vi "qTRA.vi"(0 "System no.":i32=1 min=1 max=4 step=1, 2 "Axes to query":string[](array[string]), 3 "Vector component":dbl[](array[numeric]) format="%.6f", 4 "No.of digits":i16=4, 5 "error in":errorcluster) -> (14 "Max. position":dbl[](array[numeric]) format="%.6f", 19 "error out":errorcluster)   [LabVIEW 2026]
doc: "Returns the maximum absolute position which can be reached from the current position in the given direction. The direction is defined by a vector (X, Y, Z, U, V, W) = (x, y, z, u, v, w). Softlimits are taken into account. In case the parallel kinematics positioner is in motion, an error will be set.\n\nC-887, F-206, M-8X0: Only for GCS syntax version = GCS 2.0 or higher (check with CSV?.vi. If CSV?.vi is not supported, syntax version is GCS 1.0)."
panel:
  # "Returns the maximum absolute position which can be reached from the current \nposition in the given direction. The direction is defined by a vector (X, Y, Z, U, V, W)."
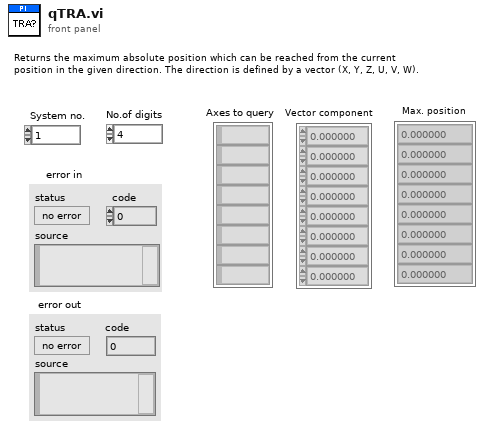
[diagram p1: front panel]
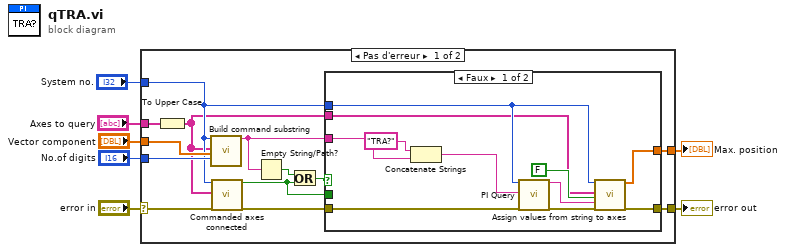
[diagram p0: block diagram]
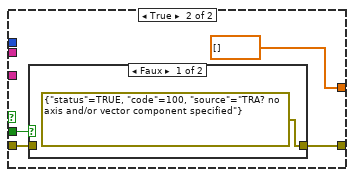
[diagram p2: hidden frame]
diagram:
  n1 = case shown="Pas d'erreur" "error in" {
    selector: "error in" -> [w14 w39]
    tunnel: "Axes to query" -> [w20 _]
    tunnel: [w16 w39] -> w6
    tunnel: "System no." -> [w12 _]
    tunnel: "Vector component" -> [w19 _]
    tunnel: "No.of digits" -> [w18 _]
    tunnel: [w17 dbl[] [] ("Values")] -> w1
    frame No Error {
      n2 = To Upper Case(1:w20) -> (0:w11:string[])
      n3 = call "Build command substring.vi"("System no."=w12, "Affected axes"=w11, "Parameters"=w19, "No. of digits"=w18) -> ("Command substring"=w15:string)  [unwired: 3 in, 12 out]
      n4 = call "Commanded axes connected.vi"("System no."=w12, "Commanded axes"=w11, "error in"=w14) -> ("Controller error"=w8:bool, "error out"=w13:errorcluster)  [unwired: 1 in, 14 out]
      n5 = Empty String/Path?(string/path=w15) -> (empty?=w10:bool)
      n6 = Or(x=w10, y=w8) -> (x .or. y?=w9:bool)
      n7 = case shown="Faux" w9 {
        tunnel: [w30 w35] -> w16
        tunnel: w13 -> [w21 w34]
        tunnel: w11 -> [w25 _]
        tunnel: w12 -> [w28 _]
        tunnel: [w29 dbl[] [] ("Values")] -> w17
        tunnel: w15 -> [w23 _]
        tunnel: w8 -> [_ w32]
        frame False {
          n8 = Concatenate Strings("TRA?", w23) -> (w22:string)
          n9 = call "PI Query.vi"("System no."=w28, "String to send"=w22, "error in"=w21) -> ("String read"=w27:string, "error out"=w31:errorcluster)  [unwired: 4 in, 11 out]
          n10 = call "Assign values from string to axes.vi"("System no."=w28, "Queried axes"=w25, "All axes queried?"=FALSE, "Input String"=w27, "error in"=w31) -> ("Values"=w29:dbl[], "error out"=w30:errorcluster)  [unwired: 4 in, 9 out]
        }
        frame True {
          n11 = case shown="Faux" w32 {
            tunnel: [errorcluster {"status"=TRUE, "code"=100, "source"="TRA? no axis and/or vector component specified"} ("error out") w37] -> w35
            tunnel: w34 -> [_ w37]
            frame False {
            }
            frame True {
            }
          }
        }
      }
    }
    frame Error {
    }
  }
  "error out" <- w6
  "Max. position" <- w1
